vi "Constructor.vi"(8 "error in (no error)":errorcluster, 11 "NYPizzaIngredientFactory in":refnum<class "NYPizzaIngredientFactory.lvclass">) -> (0 "error out":errorcluster, 3 "NYPizzaIngredientFactory out":refnum<class "NYPizzaIngredientFactory.lvclass">)   [LabVIEW 2013, in "NYPizzaIngredientFactory.lvclass"]
uses:
  NYPizzaIngredientFactory.lvclass
  ThinDough.lvclass/ThinDough/ThinDough.lvclass
  Marinara.lvclass/Marinara.lvclass
  Reggiano.lvclass/Reggiano.lvclass
  FreshClams.lvclass/FreshClams.lvclass
  NYPizzaIngredientFactory.lvclass/NYPizzaIngredientFactory.ctl
panel:
  # "紐約工廠指定紐約口味使用的食材"
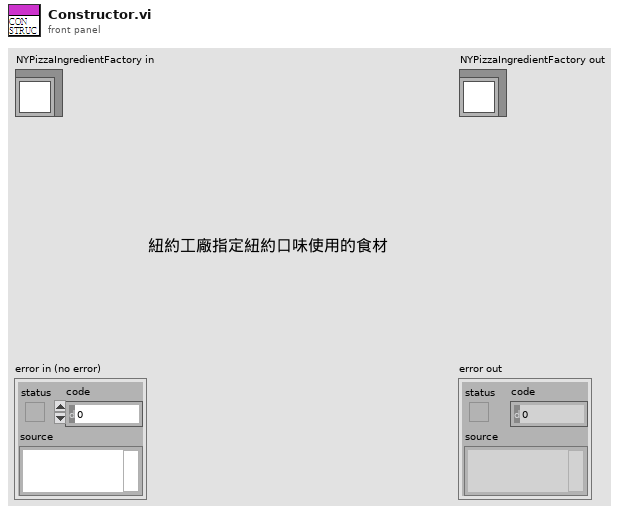
[diagram p1: front panel]
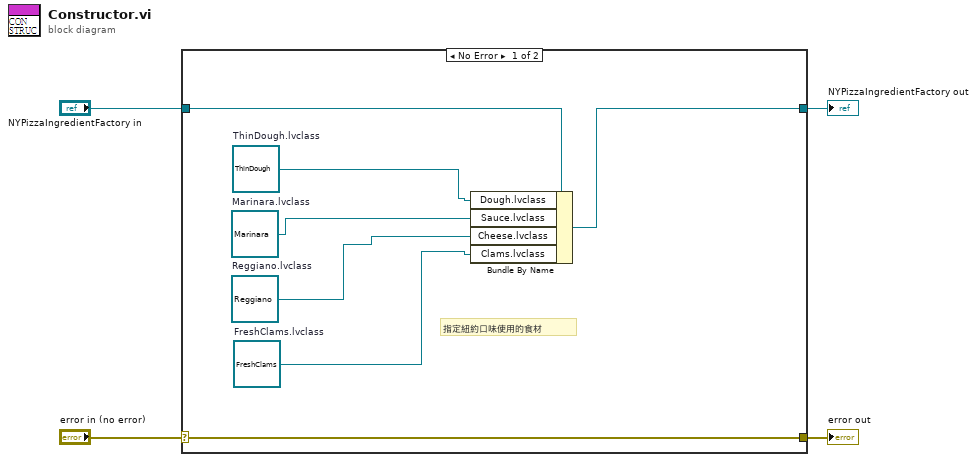
[diagram p0: block diagram]
diagram:
  n1 = case shown="No Error" "error in (no error)" {
    selector: "error in (no error)" -> [w11 w13]
    tunnel: [w11 w13] -> w3
    tunnel: [w5 w12] -> w1
    tunnel: "NYPizzaIngredientFactory in" -> [w6 w12]
    frame No Error {
      w7 = refnum<class "FreshClams.lvclass"> refnum  # FreshClams.lvclass
      w8 = refnum<class "Reggiano.lvclass"> refnum  # Reggiano.lvclass
      w9 = refnum<class "Marinara.lvclass"> refnum  # Marinara.lvclass
      w10 = refnum<class "ThinDough.lvclass"> refnum  # ThinDough.lvclass
      # "指定紐約口味使用的食材"
      n2 = Bundle By Name(cluster=w6, "Dough.lvclass"=w10, "Sauce.lvclass"=w9, "Cheese.lvclass"=w8, "Clams.lvclass"=w7) -> (w5:refnum<class "NYPizzaIngredientFactory.lvclass">)
    }
    frame Error {
    }
  }
  "error out" <- w3
  "NYPizzaIngredientFactory out" <- w1
